vi "Mcp2221 Get Last Error.vi"(0 "VID":u32=1240 format="%.0x", 5 "PID":u32=221 format="%.0x", 7 "Serial No (max 10 Char)":string, 9 "index":i32, 11 "error in (no error)":errorcluster) -> (15 "error out":errorcluster)   [LabVIEW 2020]
doc: "MCP2221_DLL_UM_API int CALLING_CONVENTION Mcp2221_GetLastError();"
uses:
  mcp2221_dll_um_x64.dll
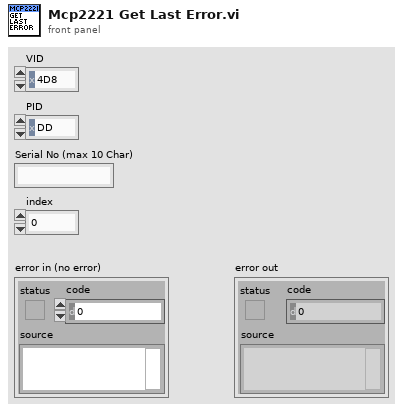
[diagram p1: front panel]
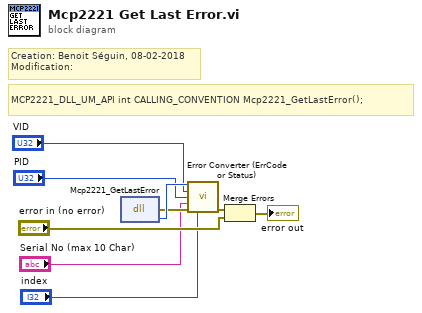
[diagram p0: block diagram]
diagram:
  # "Creation: Benoit Séguin, 08-02-2018\nModification:"
  # "MCP2221_DLL_UM_API int CALLING_CONVENTION Mcp2221_GetLastError();"
  n1 = dll-call lib="C:/Users/tuguialexand/Desktop/Licenta/MCP2221A LabVIEW library/Microchip MCP2221A_64bit/VIs/Private/mcp2221_dll_um_x64.dll" fn="Mcp2221_GetLastError"() -> (error out=w8:errorcluster, "return type"=w9:i32)  [unwired: 3 in, 1 out]
  n2 = call "Error Converter (ErrCode or Status).vi"("error code"=w9, "VID"="VID", "PID"="PID", "Serial No (max 10 Char)"="Serial No (max 10 Char)", "error in (no error)"=w8, "index"="index") -> ("error out"=w6:errorcluster)  [unwired: 9 in]
  n3 = Merge Errors(w6, "error in (no error)") -> (→"error out":errorcluster)
